vi "RenderLines.vi"(8 "No Error":errorcluster, 10 "points":T1[](array[typedef]), 11 "renderer [SDL_Renderer *]":i64) -> (0 "error out":errorcluster)   [LabVIEW 2024, in "SDL3.lvlib" / "Render.lvlib"]
doc: "<B>Summary</B>\nDraw a series of connected lines on the current rendering target at subpixel precision.\n\n<B>Thread Safety</B>\nYou may only call this function from the main thread."
uses:
  Render.lvlib
  FPoint--cluster.ctl
  Error/Error.lvlib
  Lib/SDL3-32.dll
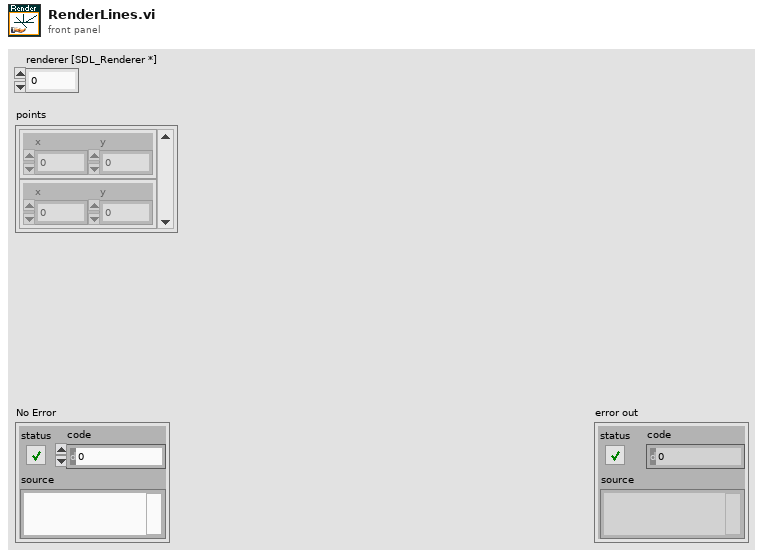
[diagram p1: front panel]
types:
  T1 = typedef "SDL3.lvlib/Render.lvlib/FPoint--cluster.ctl" = cluster{"x":sgl, "y":sgl}
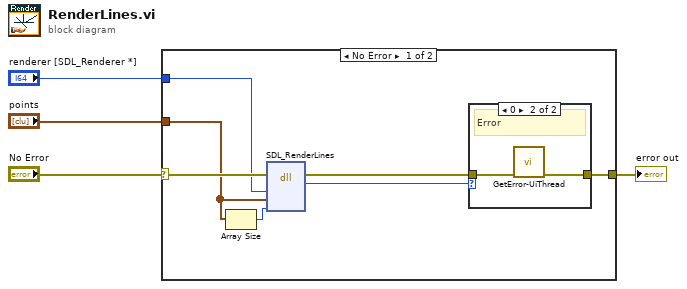
[diagram p0: block diagram]
diagram:
  n1 = case shown="No Error" "No Error" {
    selector: "No Error" -> [w11 w15]
    tunnel: [w9 w15] -> w3
    tunnel: "renderer [SDL_Renderer *]" -> [w7 _]
    tunnel: "points" -> [w6 _]
    frame No Error {
      n2 = Array Size(array=w6) -> (size(s)=w5:i32)
      n3 = dll-call lib="C:/Users/Thomas/Documents/Projects/LV-SDL3/Lib/SDL3-*.*" fn="SDL_RenderLines"(error in=w11, "renderer"=w7, "points"=w6, "count"=w5) -> (error out=w10:errorcluster, "return type"=w8:i32)  [unwired: 5 in, 1 out]
      n4 = case shown="0" w8 {
        tunnel: w10 -> [w12 w14]
        tunnel: [w12 w13] -> w9
        frame Default {
          # "Ok"
        }
        frame 0 {
          # "Error"
          n5 = call "GetError-UiThread.vi"("No Error"=w14) -> ("error out"=w13:errorcluster)  [unwired: 10 in]
        }
      }
    }
    frame Error {
    }
  }
  "error out" <- w3
